vi "01 - Acquire Analyze Present (Sequential).vi"() -> ()   [LabVIEW 2025]
uses:
  <vilib>/express/express analysis/Spectral/Block/exnSpectralBlock spectral measurements power poly.vi
  <vilib>/express/express analysis/Spectral/Block/exnSpectralBlock spectral measurements power DDT.vi
  <vilib>/express/express analysis/Spectral/XNode/ExpressSpectralMeasurementsBlockNode.xnode
  <vilib>/addons/Time Frequency Analysis/_control.llb/TFA Configure Spectrogram Indicator (Predefined Color Table).vi
  <vilib>/addons/_Advanced Signal Processing/NI_AdvSigProcTFA.lvlib
panel:
  in  "Lower Cutoff, Hz":dbl=1600.0 format="%.3p"
  in  "Acquisition Duration, sec":dbl=3.0 format="%#_13g"
  out "Time Domain":dynamicdata(graph)
  out "Power Spectrum":dynamicdata(graph)
  out "Spectrogram":dbl[][](graph)
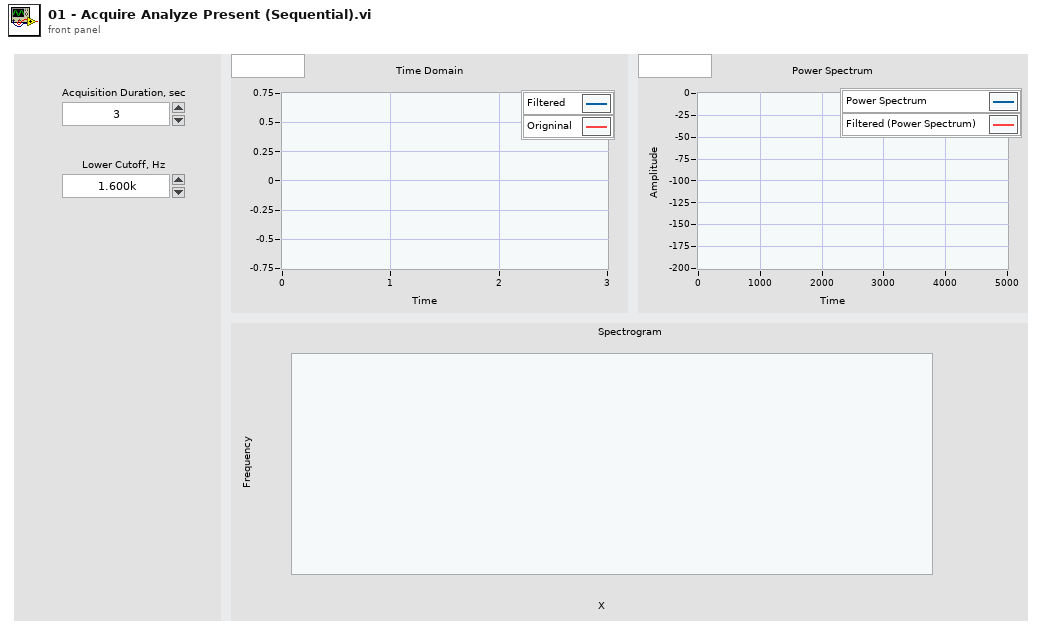
[diagram p1: front panel]
types:
  T1 = cluster{"averaging mode":u16, "weighting mode":u16, "number of averages":u32}
  T2 = cluster{"dB On (F)":bool, "unwrap phase (F)":bool, "convert to degree (F)":bool}
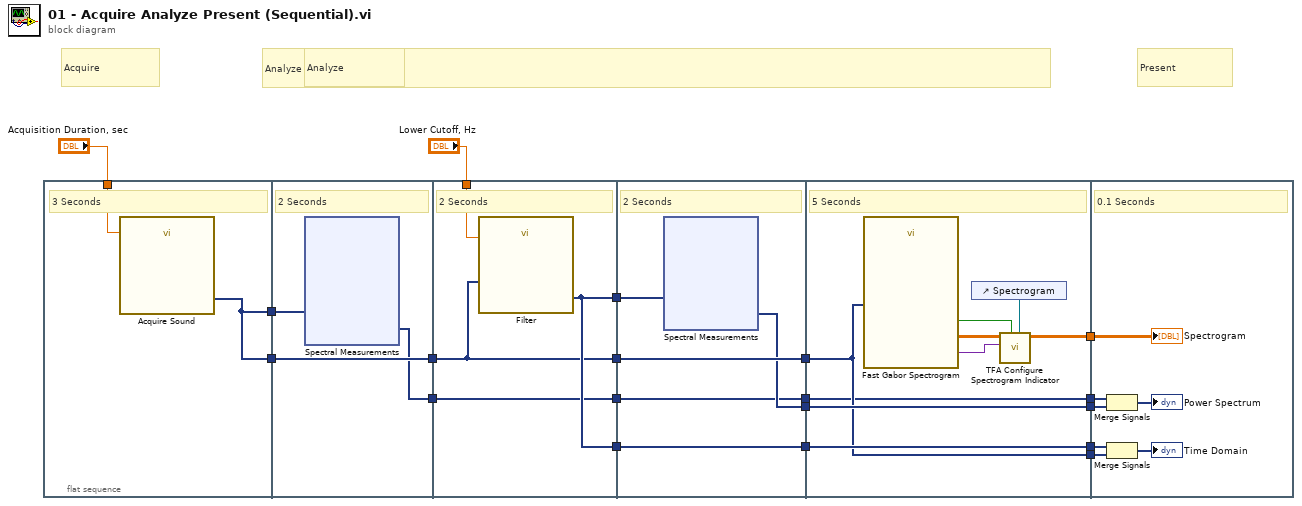
[diagram p0: block diagram]
diagram:
  # "Analyze"
  # "Present"
  # "Analyze"
  # "Acquire"
  n1 = flat-sequence {
    tunnel: "Acquisition Duration, sec" -> [w21]
    tunnel: [w20] -> w18
    tunnel: [w20] -> w16
    tunnel: w18 -> [w24]
    tunnel: [w23] -> w17
    tunnel: w16 -> [w23]
    tunnel: [w22] -> w4
    tunnel: w17 -> [w35]
    tunnel: [w36] -> w15
    tunnel: "Lower Cutoff, Hz" -> [w37]
    tunnel: [w35] -> w11
    tunnel: [w36] -> w6
    tunnel: w4 -> [w34]
    tunnel: [w34] -> w3
    tunnel: w15 -> [w42]
    tunnel: [w41] -> w12
    tunnel: w11 -> [w41]
    tunnel: [w40] -> w9
    tunnel: [w39] -> w7
    tunnel: w6 -> [w39]
    tunnel: w3 -> [w38]
    tunnel: [w38] -> w2
    tunnel: [w56] -> w14
    tunnel: w12 -> [w53]
    tunnel: [w55] -> w10
    tunnel: w9 -> [w55]
    tunnel: [w54] -> w8
    tunnel: w7 -> [w54]
    tunnel: [w53] -> w5
    tunnel: w2 -> [w52]
    tunnel: [w52] -> w1
    tunnel: w14 -> [w67]
    tunnel: w10 -> [w63]
    tunnel: w8 -> [w65]
    tunnel: w5 -> [w64]
    tunnel: w1 -> [w62]
    frame #0 {
      # "3 Seconds"
      n2 = call "Acquire Sound"("Duration (s)"=w21) -> ("Data"=w20:dynamicdata)  [unwired: 17 in, 1 out]
    }
    frame #1 {
      # "2 Seconds"
      n3 = xnode "Spectral Measurements"("Signals"=w24) -> ("Power Spectrum"=w22:dynamicdata)  [unwired: 1 in, 1 out]
    }
    frame #2 {
      # "2 Seconds"
      n4 = call "Filter"("Lower Cut-Off"=w37, "Signal"=w35) -> ("Filtered Signal"=w36:dynamicdata)  [unwired: 8 in, 1 out]
    }
    frame #3 {
      # "2 Seconds"
      n5 = xnode "Spectral Measurements"("Signals"=w42) -> ("Power Spectrum"=w40:dynamicdata)  [unwired: 1 in, 1 out]
    }
    frame #4 {
      # "5 Seconds"
      n6 = call "Fast Gabor Spectrogram"("Signal"=w53) -> ("Scale Info"=w60:variant, "Spectrogram"=w57:dbl[][], "dB"=w59:bool)  [unwired: 6 in, 2 out]
      n7 = control-ref of="Spectrogram"() -> (w58:refnum<vi>)
      n8 = call-poly <vilib>:"TFA Configure Spectrogram Indicator.vi"("reference of TF spectrogram indicator"=w58, "dB on? (F)"=w59, "scale info"=w60, "spectrogram"=w57) -> ("TF spectrogram indicator"=w56:dbl[][])  [unwired: 6 in, 1 out]
    }
    frame #5 {
      # "0.1 Seconds"
      n9 = Merge Signals(w62, w63) -> (→"Power Spectrum":dynamicdata)
      n10 = Merge Signals(w65, w64) -> (→"Time Domain":dynamicdata)
      "Spectrogram" <- w67
    }
  }
